vi "Discover Unique Names of Dependencies.vi"(0 "VIP In":refnum<class "VIP.lvclass">) -> (4 "VIP Out":refnum<class "VIP.lvclass">)   [LabVIEW 2017, in "CL_G3_VIComponentBuilder.lvlib" / "VIP.lvclass"]
doc: "Parses the VI Package Build spec to get all of the vi packages that this vi package depends on."
uses:
  VIP.lvclass
  C:/Tool Chain Support/Software Module Builder/Source/Exports/Exports/Export.lvclass
  Exports/Export.lvclass/Export.ctl
  Exports/Accessors/Read Export Build Specification.vi
  Exports/Accessors/Read Export Operation Errors.vi
  <vilib>/xml/Close Reference(Node).vi
  <vilib>/xml/Close Reference(NdList).vi
  Exports/Accessors/Write Dependencies' Unique Names.vi
  Exports/Export.lvclass
  <resource>/objmgr/DOMUserDefRef.rc
  <vilib>/xml/NI_XML.lvlib
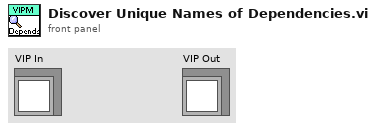
[diagram p1: front panel]
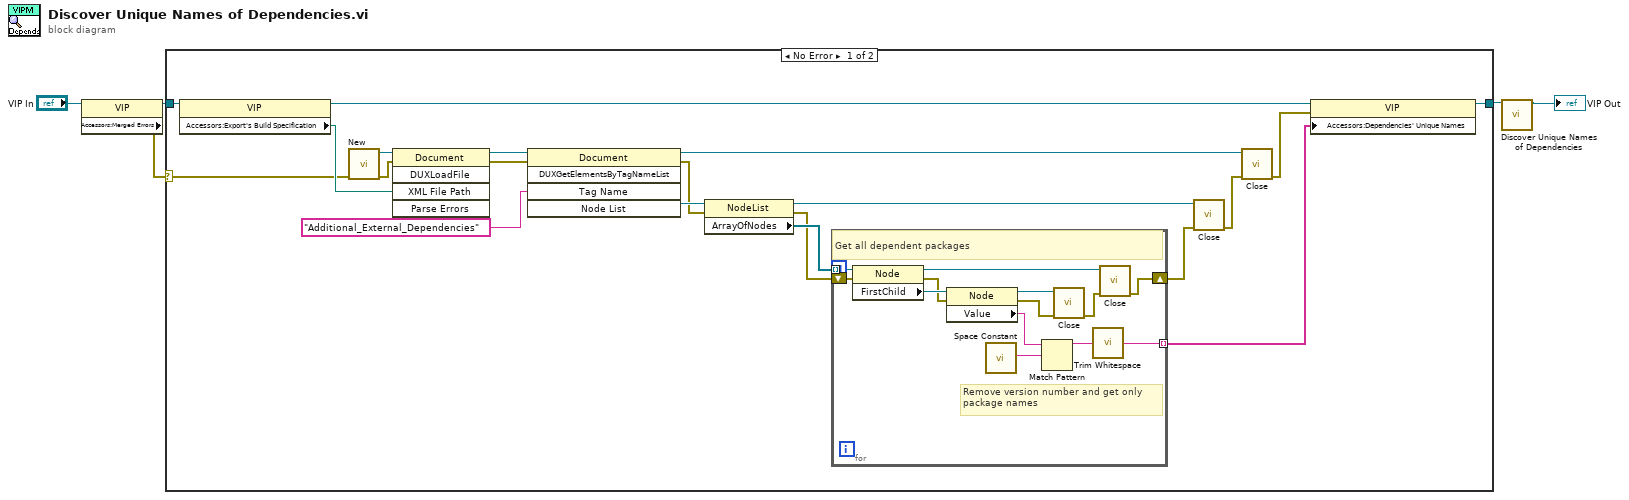
[diagram p0: block diagram]
diagram:
  n1 = property class="VIP"(reference="VIP In") -> (reference out=w1:refnum<class "VIP.lvclass">, "Accessors:Merged Errors"=w2:errorcluster)  [unwired: 1 in, 1 out]
  n2 = case shown="No Error" w2 {
    selector: w2 -> [w10 _]
    tunnel: [w6 w39] -> w5
    tunnel: w1 -> [w11 w39]
    frame No Error {
      n3 = property class="VIP"(reference=w11) -> (reference out=w9:refnum<class "VIP.lvclass">, "Accessors:Export's Build Specification"=w14:path)  [unwired: 1 in, 1 out]
      n4 = call <vilib>:"New.vi"("error in (no error)"=w10) -> ("error out"=w24:errorcluster, "DOM document out"=w25:refnum<k20>)  [unwired: 7 in]
      n5 = invoke class="Document" method="DUXLoadFile"(reference=w25, error in=w24, "XML File Path"=w14) -> (reference out=w13:refnum<k20>, error out=w12:errorcluster)  [unwired: 2 in, 3 out]
      n6 = invoke class="Document" method="DUXGetElementsByTagNameList"(reference=w13, error in=w12, "Tag Name"="Additional_External_Dependencies") -> (reference out=w23:refnum<k20>, error out=w18:errorcluster, "Node List"=w22:refnum<k20>)  [unwired: 2 in, 2 out]
      n7 = property class="NodeList"(reference=w22, error in=w18) -> (reference out=w16:refnum<k20>, error out=w17:errorcluster, "ArrayOfNodes"=w19:refnum<k20>[])
      n8 = for {
        tunnel: [w26] -> w8 mode=indexing
        tunnel: w19 -> [w38] mode=indexing
        shift-right: [w30] -> w15
        shift-left: w17 -> [w36]
        # "Remove version number and get only\npackage names"
        # "Get all dependent packages"
        n9 = property class="Node"(reference=w38, error in=w36) -> (reference out=w32:refnum<k20>, error out=w33:errorcluster, "FirstChild"=w37:refnum<k20>)
        n10 = property class="Node"(reference=w37, error in=w33) -> (reference out=w34:refnum<k20>, error out=w35:errorcluster, "Value"=w29:string)
        n11 = call <vilib>:"Space Constant.vi"() -> ("String"=w27:string)
        n12 = Match Pattern(string=w29, regular expression=w27) -> (before substring=w28:string)  [unwired: 1 in, 3 out]
        n13 = call-poly <vilib>:"Close.vi"("error in (no error)"=w35, "node"=w34) -> ("error out"=w31:errorcluster)  [unwired: 7 in]
        n14 = call <vilib>:"Trim Whitespace.vi"("string"=w28) -> ("trimmed string"=w26:string)  [unwired: 1 in]
        n15 = call-poly <vilib>:"Close.vi"("error in (no error)"=w31, "node"=w32) -> ("error out"=w30:errorcluster)  [unwired: 7 in]
      }
      n16 = call-poly <vilib>:"Close.vi"("error in (no error)"=w15, "node list"=w16) -> ("error out"=w20:errorcluster)  [unwired: 7 in]
      n17 = call-poly <vilib>:"Close.vi"("error in (no error)"=w20, "node"=w23) -> ("error out"=w7:errorcluster)  [unwired: 7 in]
      n18 = property class="VIP"(reference=w9, error in=w7, "Accessors:Dependencies' Unique Names"=w8) -> (reference out=w6:refnum<class "VIP.lvclass">)  [unwired: 1 out]
    }
    frame Error {
    }
  }
  n19 = call-parent "Discover Unique Names of Dependencies.vi"("Export In"=w5) -> ("Export Out"=→"VIP Out":refnum<class "VIP.lvclass">)  [unwired: 14 in]
